vi "aft_Check_LVFPGA_Installed.vi"(8 "error in (no error)":errorcluster) -> (0 "error out":errorcluster)   [LabVIEW 2017, in "NI_AdaptiveFilter.lvlib"]
uses:
  <vilib>/addons/Adaptive Filters/NI_AdaptiveFilter.lvlib
  <vilib>/addons/Adaptive Filters/Utilities/AFT Errors.ctl
  <vilib>/registry/registry.llb/Registry RtKey.ctl
  <vilib>/registry/registry.llb/Registry SAM.ctl
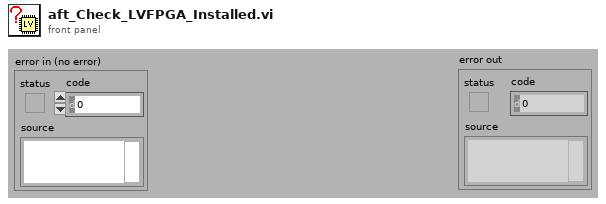
[diagram p1: front panel]
types:
  T1 = typedef "Registry SAM.ctl" = enum32{"KEY_QUERY_VALUE", "KEY_SET_VALUE", "KEY_CREATE_SUB_KEY", "KEY_ENUMERATE_SUB_KEYS", "KEY_NOTIFY", "KEY_CREATE_LINK", "KEY_READ", "KEY_WRITE", "KEY_ALL_ACCESS", "KEY_READ | KEY_WRITE"}
  T2 = typedef "Registry RtKey.ctl" = enum32{"HKEY_CLASSES_ROOT", "HKEY_CURRENT_USER", "HKEY_LOCAL_MACHINE", "HKEY_USERS", "HKEY_PERFORMANCE_DATA", "HKEY_CURRENT_CONFIG", "HKEY_DYN_DATA"}
  T3 = typedef "NI_AdaptiveFilter.lvlib/AFT Errors.ctl" = i32
  T4 = typedef "Registry refnum.ctl" = refnum<k1>
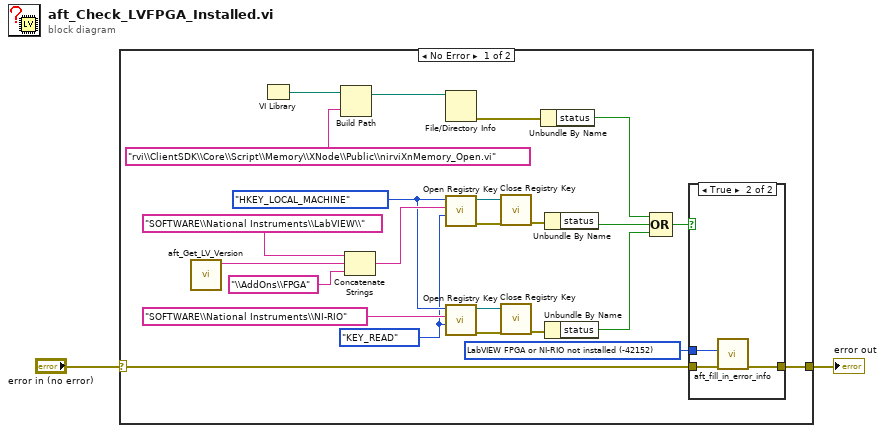
[diagram p0: block diagram]
diagram:
  n1 = case shown="No Error" "error in (no error)" {
    selector: "error in (no error)" -> [w6 w31]
    tunnel: [w7 w31] -> w2
    frame No Error {
      w8 = Registry_SAM."KEY_READ" ("security access mask (KEY_READ | KEY_WRITE)")
      w11 = Registry_RtKey."HKEY_LOCAL_MACHINE" ("root key (HKEY_LOCAL_MACHINE)")
      w3 = T3 -42152 items=["No errors"=0, "No valid FPGA target"=-42150, "Invalid filter configurations"=-42151, "LabVIEW FPGA or NI-RIO not installed"=-42152, "File exists on disk"=-42153, "File exists in memory"=-42154] ("AFT errors")
      n2 = call <vilib>:"aft_Get_LV_Version.vi"() -> ("LV version"=w4:string)  [unwired: 11 out]
      n3 = VI Library() -> (path=w19:path)
      n4 = Build Path(base path=w19, name or relative path="rvi\\ClientSDK\\Core\\Script\\Memory\\XNode\\Public\\nirviXnMemory_Open.vi") -> (appended path=w16:path)
      n5 = Concatenate Strings("SOFTWARE\\National Instruments\\LabVIEW\\" ("subkey"), w4, "\\AddOns\\FPGA" ("subkey")) -> (w23:string)
      n6 = File/Directory Info(path=w16) -> (error out=w15:errorcluster)  [unwired: 1 in, 6 out]
      n7 = call <vilib>:"Open Registry Key.vi"("security access mask (KEY_READ | KEY_WRITE)"=w8, "subkey"=w23, "root key (HKEY_LOCAL_MACHINE)"=w11) -> ("error out"=w26:errorcluster, "refnum out"=w25:T4)  [unwired: 1 in, 6 out]
      n8 = call <vilib>:"Open Registry Key.vi"("security access mask (KEY_READ | KEY_WRITE)"=w8, "subkey"="SOFTWARE\\National Instruments\\NI-RIO", "root key (HKEY_LOCAL_MACHINE)"=w11) -> ("error out"=w12:errorcluster, "refnum out"=w13:T4)  [unwired: 1 in, 6 out]
      n9 = call <vilib>:"Close Registry Key.vi"("error in (no error)"=w26, "refnum"=w25) -> ("error out"=w24:errorcluster)  [unwired: 5 out]
      n10 = call <vilib>:"Close Registry Key.vi"("error in (no error)"=w12, "refnum"=w13) -> ("error out"=w14:errorcluster)  [unwired: 5 out]
      n11 = Unbundle By Name(w15) -> ("status"=w17:bool)
      n12 = Unbundle By Name(w24) -> ("status"=w22:bool)
      n13 = Unbundle By Name(w14) -> ("status"=w9:bool)
      n14 = Compound Arithmetic op=OR(w17, w22, w9) -> (w5:bool)
      n15 = case shown="True" w5 {
        tunnel: [w27 w29] -> w7
        tunnel: w6 -> [w27 w30]
        tunnel: w3 -> [_ w28]
        frame False {
        }
        frame True {
          n16 = call <vilib>:"aft_fill_in_error_info.vi"("error in"=w30, "status code"=w28) -> ("error out"=w29:errorcluster)  [unwired: 2 in, 7 out]
        }
      }
    }
    frame Error {
    }
  }
  "error out" <- w2
